vi "usb650.vi"() -> ()   [LabVIEW 2011]
panel:
  out "Integration Time 2":i32
  in  "stop":bool
  in  "Run/Pause":bool
  in  "Integration Time":i32
  out "Num Spectrometers":i32
  out "XY Graph":cluster{"Y":dbl[], "Y":dbl[]}[](graph)
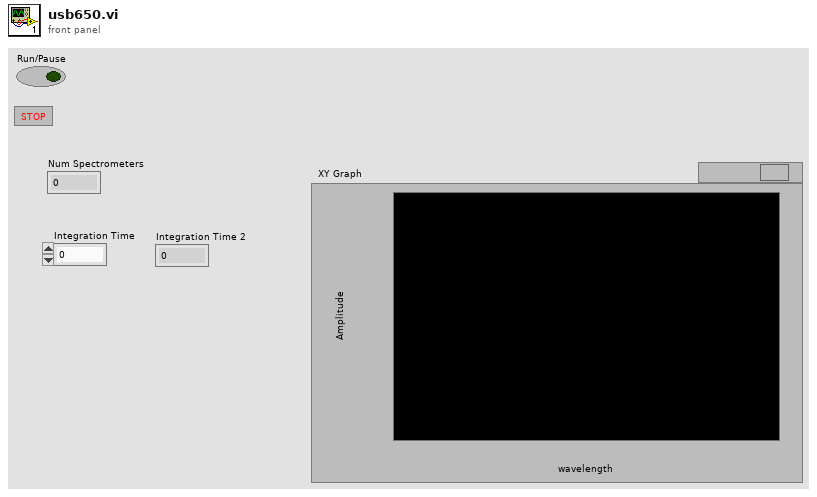
[diagram p1: front panel]
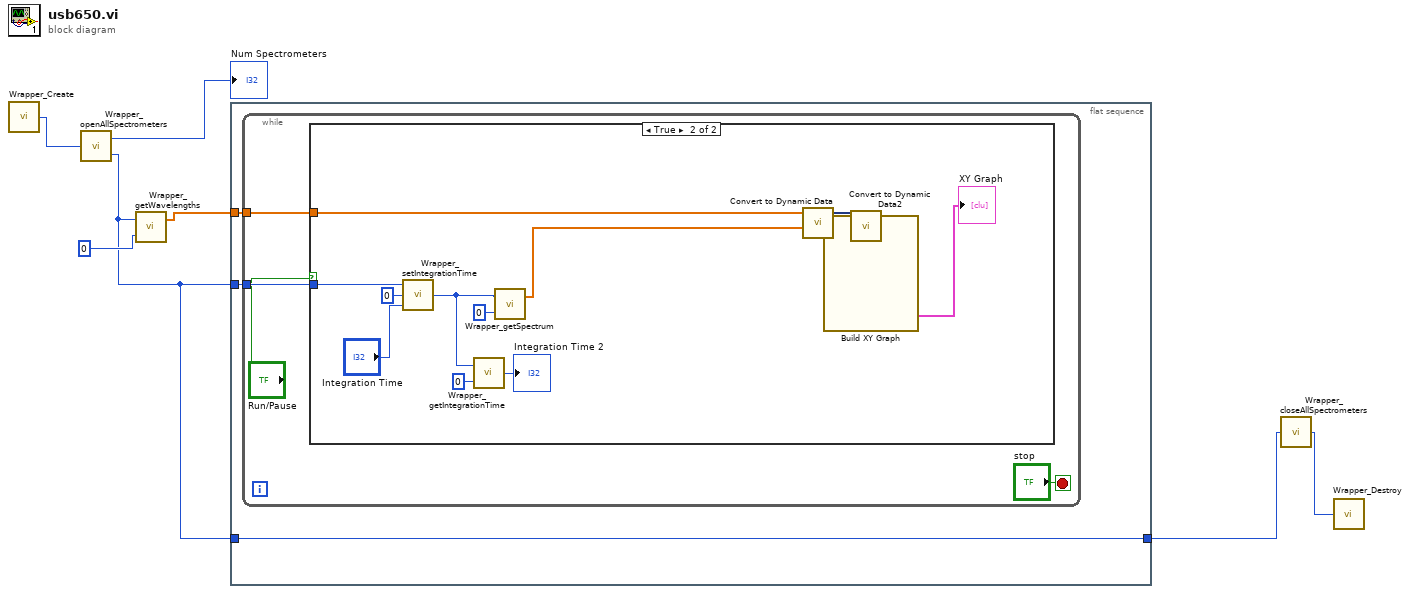
[diagram p0: block diagram]
diagram:
  n1 = call "Wrapper_Create.vi"() -> ("Wrapper"=w7:u32)
  n2 = call "Wrapper_openAllSpectrometers.vi"("Wrapper In"=w7) -> ("Number of Spectrometers"=→"Num Spectrometers":i32, "Wrapper Out"=w2:u32)
  n3 = call "Wrapper_getWavelengths.vi"("Index"=0, "Wrapper"=w2) -> ("WL Values"=w5:dbl[])  [unwired: 1 out]
  n4 = flat-sequence {
    tunnel: w5 -> [w10]
    tunnel: w2 -> [w9]
    tunnel: [w8] -> w1
    tunnel: w2 -> [w8]
    frame #0 {
      n5 = while {
        tunnel: w10 -> [w14]
        tunnel: w9 -> [w13]
        stop <- "stop" stop-if-true
        n6 = case shown="True" "Run/Pause" {
          tunnel: w14 -> [_ w25]
          tunnel: w13 -> [_ w18]
          frame False {
          }
          frame True {
            n7 = call "Wrapper_setIntegrationTime.vi"("Integration Time"="Integration Time", "Index"=0, "Wrapper In"=w18) -> ("Wrapper Out"=w17:u32)
            n8 = call "Wrapper_getIntegrationTime.vi"("Index"=0, "Wrapper"=w17) -> ("Integration Time"=→"Integration Time 2":i32)
            n9 = call "Wrapper_getSpectrum.vi"("Index"=0, "Wrapper"=w17) -> ("Spectrum Values"=w23:dbl[])  [unwired: 1 out]
            n10 = call "Convert to Dynamic Data"("Array"=w25) -> ("Dynamic Data Type"=w24:dynamicdata)  [unwired: 3 in]
            n11 = call "Convert to Dynamic Data2"("Array"=w23) -> ("Dynamic Data Type"=w22:dynamicdata)  [unwired: 3 in]
            n12 = call "Build XY Graph"("Y Input"=w22, "X Input"=w24) -> ("XY Graph"=→"XY Graph":cluster{"Y":dbl[], "Y":dbl[]}[])  [unwired: 3 in, 6 out]
          }
        }
      }
    }
  }
  n13 = call "Wrapper_closeAllSpectrometers.vi"("Wrapper In"=w1) -> ("Wrapper Out"=w3:u32)
  n14 = call "Wrapper_Destroy.vi"("Wrapper"=w3) -> ()
